vi "test Import Export SLSC Switch CD.vi"(8 "error in (no error)":errorcluster, 11 "TestCase in":refnum<class "SLSC Switch Scripting Unit Tests.lvclass">) -> (0 "error out":errorcluster, 3 "TestCase out":refnum<class "SLSC Switch Scripting Unit Tests.lvclass">)   [LabVIEW 2017, in "SLSC Switch Scripting Unit Tests.lvclass"]
uses:
  SLSC Switch Scripting Unit Tests.lvclass
  Shared/Endpoint Configuration Cluster.ctl
  Shared/Endpoint Configuration Enum.ctl
  SLSC Switch Scripting Unit Tests.lvclass/SLSC Switch Scripting Unit Tests.ctl
  Custom Device/Find All SLSC Switch Custom Devices.vi
  <userlib>/_OpenG.lib/file/file.llb/Append Path to Root if Relative - Scalar__ogtk.vi
  <vilib>/addons/_JKI Toolkits/VI Tester/TestCase.llb/TestCase.lvclass
  SLSC Switch Scripting.lvlib
  Shared/SLSC Switch Shared.lvlib
  niveristand-custom-device-testing-tools/VeriStandTestUtilities/VeriStandTestUtilities.lvlib
  C:/Program Files (x86)/National Instruments/LabVIEW 2017/vi.lib/addons/_JKI Toolkits/VI Tester/TestCase.llb/TestCase.lvclass
panel:
  in  "Save?":bool
  out "Output Filename":string
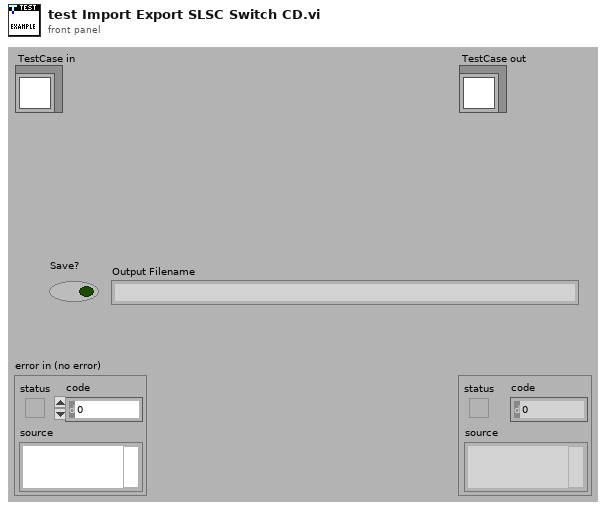
[diagram p1: front panel]
types:
  T1 = enum16{"open", "replace", "create", "open or create", "replace or create", "replace or create with confirmation"}
  T2 = typedef "SLSC Switch Shared.lvlib/Endpoint Configuration Cluster.ctl" = cluster{"Endpoint":string, "Configuration":T3}
  T3 = typedef "SLSC Switch Shared.lvlib/Endpoint Configuration Enum.ctl" = enum16{"Load", "Source", "Configuration"}
  T4 = typedef "Custom Device API.lvlib/Custom Device Item Ref.ctl" = u64
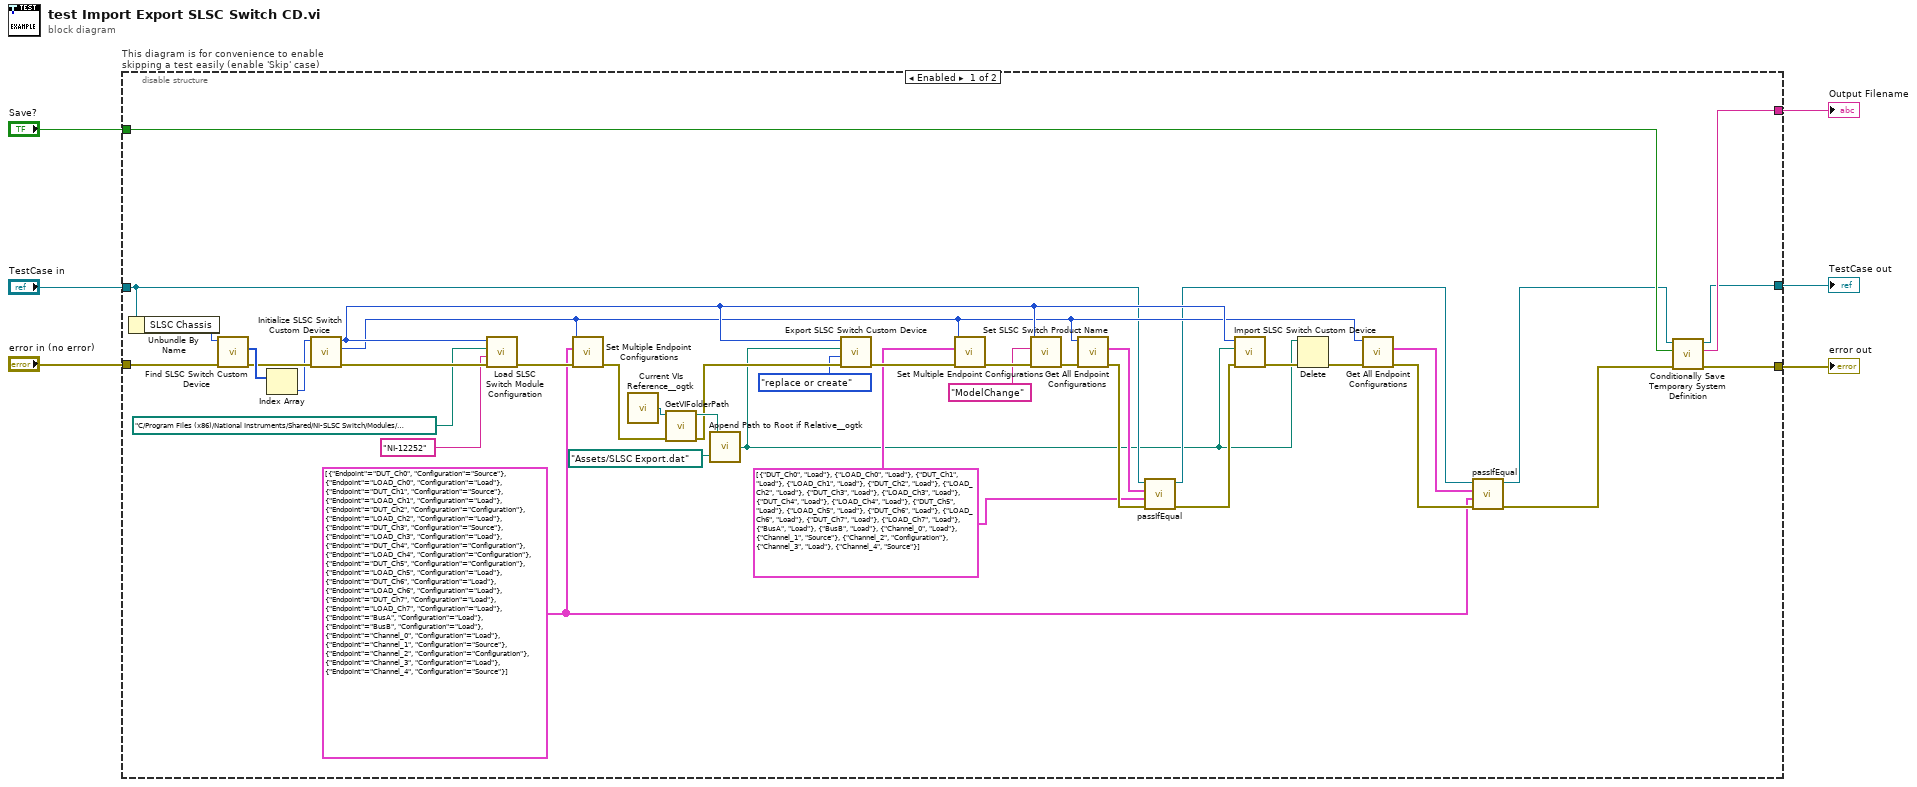
[diagram p0: block diagram]
diagram:
  n1 = disable-structure "This diagram is for convenience to enable skipping a test easily (enable 'Skip' case)" shown="Enabled" {
    disable-tunnel: "TestCase in" -> [w13 w49]
    disable-tunnel: [w43 w47] -> w3
    disable-tunnel: [w44 w48] -> w5
    disable-tunnel: "error in (no error)" -> [w37 w46]
    disable-tunnel: [w45 _] -> w2
    disable-tunnel: "Save?" -> [w42 _]
    frame Enabled {
      w10 = T2[] [{"Endpoint"="DUT_Ch0", "Configuration"=enum."Load"}, {"Endpoint"="LOAD_Ch0", "Configuration"=enum."Load"}, {"Endpoint"="DUT_Ch1", "Configuration"=enum."Load"}, {"Endpoint"="LOAD_Ch1", "Configuration"=enum."Load"}, {"Endpoint"="DUT_Ch2", "Configuration"=enum."Load"}, {"Endpoint"="LOAD_Ch2", "Configuration"=enum."Load"}, {"Endpoint"="DUT_Ch3", "Configuration"=enum."Load"}, {"Endpoint"="LOAD_Ch3", "Configuration"=enum."Load"}, {"Endpoint"="DUT_Ch4", "Configuration"=enum."Load"}, {"Endpoint"="LOAD_Ch4", "Configuration"=enum."Load"}, {"Endpoint"="DUT_Ch5", "Configuration"=enum."Load"}, {"Endpoint"="LOAD_Ch5", "Configuration"=enum."Load"}, {"Endpoint"="DUT_Ch6", "Configuration"=enum."Load"}, {"Endpoint"="LOAD_Ch6", "Configuration"=enum."Load"}, {"Endpoint"="DUT_Ch7", "Configuration"=enum."Load"}, {"Endpoint"="LOAD_Ch7", "Configuration"=enum."Load"}, {"Endpoint"="BusA", "Configuration"=enum."Load"}, {"Endpoint"="BusB", "Configuration"=enum."Load"}, {"Endpoint"="Channel_0", "Configuration"=enum."Load"}, {"Endpoint"="Channel_1", "Configuration"=enum."Source"}, {"Endpoint"="Channel_2", "Configuration"=enum."Configuration"}, {"Endpoint"="Channel_3", "Configuration"=enum."Load"}, {"Endpoint"="Channel_4", "Configuration"=enum."Source"}] ("Array")
      w23 = T2[] [{"Endpoint"="DUT_Ch0", "Configuration"=enum."Source"}, {"Endpoint"="LOAD_Ch0", "Configuration"=enum."Load"}, {"Endpoint"="DUT_Ch1", "Configuration"=enum."Source"}, {"Endpoint"="LOAD_Ch1", "Configuration"=enum."Load"}, {"Endpoint"="DUT_Ch2", "Configuration"=enum."Configuration"}, {"Endpoint"="LOAD_Ch2", "Configuration"=enum."Load"}, {"Endpoint"="DUT_Ch3", "Configuration"=enum."Source"}, {"Endpoint"="LOAD_Ch3", "Configuration"=enum."Load"}, {"Endpoint"="DUT_Ch4", "Configuration"=enum."Configuration"}, {"Endpoint"="LOAD_Ch4", "Configuration"=enum."Configuration"}, {"Endpoint"="DUT_Ch5", "Configuration"=enum."Configuration"}, {"Endpoint"="LOAD_Ch5", "Configuration"=enum."Load"}, {"Endpoint"="DUT_Ch6", "Configuration"=enum."Load"}, {"Endpoint"="LOAD_Ch6", "Configuration"=enum."Load"}, {"Endpoint"="DUT_Ch7", "Configuration"=enum."Load"}, {"Endpoint"="LOAD_Ch7", "Configuration"=enum."Load"}, {"Endpoint"="BusA", "Configuration"=enum."Load"}, {"Endpoint"="BusB", "Configuration"=enum."Load"}, {"Endpoint"="Channel_0", "Configuration"=enum."Load"}, {"Endpoint"="Channel_1", "Configuration"=enum."Source"}, {"Endpoint"="Channel_2", "Configuration"=enum."Configuration"}, {"Endpoint"="Channel_3", "Configuration"=enum."Load"}, {"Endpoint"="Channel_4", "Configuration"=enum."Source"}] ("Array")
      n2 = Unbundle By Name(w13) -> ("SLSC Chassis"=w38:u64)
      n3 = call-poly "Find SLSC Switch Custom Device.vi"("error in (no error)"=w37, "SLSC Chassis Ref"=w38) -> ("error out"=w40:errorcluster, "SLSC Switch Custom Device Ref IDs"=w41:T4[])  [unwired: 7 in, 1 out]
      n4 = Index Array(array=w41) -> (element=w39:T4)  [unwired: 1 in]
      n5 = call "Initialize SLSC Switch Custom Device.vi"("error in (no error)"=w40, "SLSC Switch Custom Device Ref in"=w39) -> ("error out"=w27:errorcluster, "Endpoint Configuration Section Ref"=w16:T4, "SLSC Switch Custom Device Ref out"=w19:T4)  [unwired: 7 in]
      n6 = call "Load SLSC Switch Module Configuration.vi"("error in"=w27, "product name"="NI-12252" ("Model"), "switches JSON file"=path "C:/Program Files (x86)/National Instruments/Shared/NI-SLSC Switch/Modules/SLSC-12252-switches.json", "SLSC Switch Custom Device Ref in"=w19) -> ("error out"=w26:errorcluster)  [unwired: 6 in, 1 out]
      n7 = call "Set Multiple Endpoint Configurations.vi"("error in (no error)"=w26, "Endpoint Configurations"=w23, "Endpoint Configuration Section Ref in"=w16) -> ("error out"=w22:errorcluster)  [unwired: 7 in, 1 out]
      n8 = call <userlib>:"Current VIs Reference__ogtk.vi"() -> ("Current VI's reference"=w36:refnum<vi>)  [unwired: 5 in]
      n9 = call "GetVIFolderPath.vi"("error in (no error)"=w22, "VI Reference in"=w36) -> ("error out"=w33:errorcluster, "VI Folder Path out"=w35:path)  [unwired: 8 in]
      n10 = call-poly <userlib>:"Append Path to Root if Relative__ogtk.vi"("Absolute or Relative Path"=path "Assets/SLSC Export.dat", "Root Path"=w35) -> ("Absolute or Appended Path"=w7:path)
      n11 = call "Export SLSC Switch Custom Device.vi"("error in (no error)"=w33, "operation"=T1."replace or create", "datalog path (use dialog)"=w7, "SLSC Switch Custom Device Ref in"=w19) -> ("error out"=w21:errorcluster)  [unwired: 6 in, 1 out]
      n12 = call "Set Multiple Endpoint Configurations.vi"("error in (no error)"=w21, "Endpoint Configurations"=w10, "Endpoint Configuration Section Ref in"=w16) -> ("error out"=w20:errorcluster)  [unwired: 7 in, 1 out]
      n13 = call "Set SLSC Switch Product Name.vi"("error in (no error)"=w20, "product name"="ModelChange" ("Model"), "SLSC Switch Custom Device Ref in"=w19) -> ("error out"=w17:errorcluster)  [unwired: 7 in, 1 out]
      n14 = call "Get All Endpoint Configurations.vi"("error in (no error)"=w17, "Endpoint Configuration Section Ref in"=w16) -> ("error out"=w15:errorcluster, "All Endpoint Configurations"=w11:T2[])  [unwired: 7 in, 1 out]
      n15 = call-dynamic "passIfEqual.vi"("error in (no error)"=w15, "y"=w10, "x"=w11, "TestCase in"=w13) -> ("error out"=w14:errorcluster, "TestCase out"=w12:refnum<class "SLSC Switch Scripting Unit Tests.lvclass">)  [unwired: 6 in]
      n16 = call "Import SLSC Switch Custom Device.vi"("error in (no error)"=w14, "datalog path (use dialog)"=w7, "SLSC Switch Custom Device Ref in"=w19) -> ("error out"=w9:errorcluster)  [unwired: 7 in, 1 out]
      n17 = Delete(path (use dialog)=w7, error in=w9) -> (error out=w8:errorcluster)  [unwired: 3 in, 2 out]
      n18 = call "Get All Endpoint Configurations.vi"("error in (no error)"=w8, "Endpoint Configuration Section Ref in"=w16) -> ("error out"=w30:errorcluster, "All Endpoint Configurations"=w29:T2[])  [unwired: 7 in, 1 out]
      n19 = call-dynamic "passIfEqual.vi"("error in (no error)"=w30, "y"=w23, "x"=w29, "TestCase in"=w12) -> ("error out"=w28:errorcluster, "TestCase out"=w31:refnum<class "SLSC Switch Scripting Unit Tests.lvclass">)  [unwired: 6 in]
      n20 = call "Conditionally Save Temporary System Definition.vi"("error in (no error)"=w28, "Save?"=w42, "Test Case"=w31) -> ("error out"=w44:errorcluster, "filename"=w45:string, "Test Case"=w43:refnum<class "SLSC Switch Scripting Unit Tests.lvclass">)  [unwired: 6 in]
    }
    frame Disabled {
      # "skip test result while test is under development"
      n21 = call <vilib>:"skip.vi"("error in (no error)"=w46, "TestCase in"=w49) -> ("error out"=w48:errorcluster, "TestCase out"=w47:refnum<class "SLSC Switch Scripting Unit Tests.lvclass">)  [unwired: 8 in]
    }
  }
  "error out" <- w5
  "TestCase out" <- w3
  "Output Filename" <- w2
